vi "ELVIS III v1.0 Configure UART.vi"(7 "Reserve?":bool, 8 "error in (no error)":errorcluster, 10 "VISA resource name in":refnum<visa-resource-name>, 11 "myRIO FPGA Ref":T1) -> (0 "error out":errorcluster)   [LabVIEW 2021]
uses:
  <vilib>/myRIO/Common/Instrument Driver Framework/Utilities/typedefs/Generic FPGA Reference.ctl
  <vilib>/myRIO/Common/Instrument Driver Framework/ELVIS III v1.0/UART/typedefs/ELVIS III v1.0 UART Channels FPGA Reference.ctl
  <vilib>/rvi/errors/niLvFpgaAdjustHostInterfaceError.vi
  <vilib>/rvi/interface/nirviReadWriteControl/nirviReadWriteControl.xnode
  <vilib>/rvi/interface/Simulation/niFpgaSimulationCallBeginRW.vi
  NiFpgaLv.dll
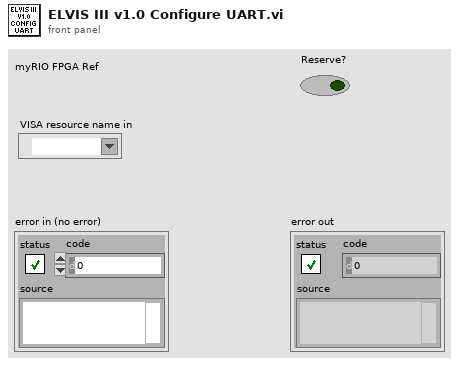
[diagram p1: front panel]
types:
  T1 = typedef "Generic FPGA Reference.ctl" = refnum<k20>
  T2 = typedef "ELVIS III v1.0 UART Channels FPGA Reference.ctl" = refnum<k20>
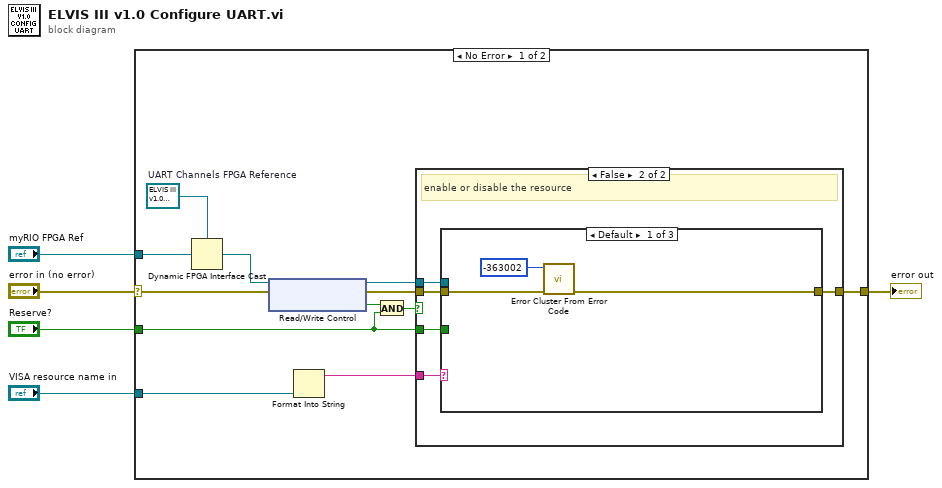
[diagram p0: block diagram]
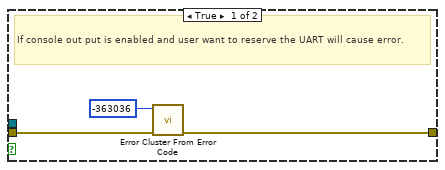
[diagram p2: hidden frame]
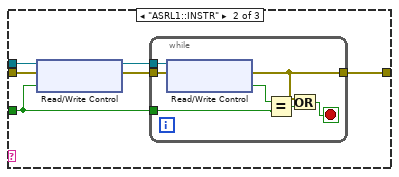
[diagram p3: hidden frame]
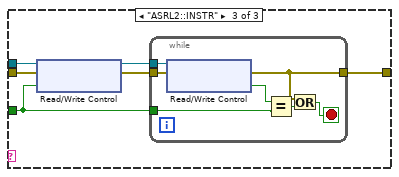
[diagram p4: hidden frame]
diagram:
  n1 = case shown="No Error" "error in (no error)" {
    selector: "error in (no error)" -> [w11 w55]
    tunnel: "myRIO FPGA Ref" -> [w17 _]
    tunnel: "VISA resource name in" -> [w9 _]
    tunnel: [w14 w55] -> w3
    tunnel: "Reserve?" -> [w7 _]
    frame No Error {
      w16 = T2 refnum  # UART Channels FPGA Reference
      n2 = Dynamic FPGA Interface Cast(Session In=w16, Type=w17) -> (Session Out=w13:T2)
      n3 = xnode "Read/Write Control"("FPGA VI Reference In"=w13, "error in"=w11) -> ("FPGA VI Reference Out"=w12:T2, "error out"=w10:errorcluster, "CONSOLE.ENA"=w8:bool)
      n4 = Format Into String(w9) -> (resulting string=w15:string)  [unwired: 3 in, 1 out]
      n5 = And(x=w8, y=w7) -> (x .and. y?=w6:bool)
      n6 = case shown="False" w6 {
        tunnel: w15 -> [_ w25]
        tunnel: [w18 w24] -> w14
        tunnel: w7 -> [_ w23]
        tunnel: w12 -> [_ w22]
        tunnel: w10 -> [w19 w21]
        frame True {
          # "If console out put is enabled and user want to reserve the UART will cause error."
          n7 = call <vilib>:"Error Cluster From Error Code.vi"("error in (no error)"=w19, "error code (0)"=-363036) -> ("error out"=w18:errorcluster)  [unwired: 7 in]
        }
        frame False {
          # "enable or disable the resource"
          n8 = case shown="Default" w25 {
            tunnel: w21 -> [w27 w34 w47]
            tunnel: [w26 w30 w43] -> w24
            tunnel: w23 -> [_ w31 w44]
            tunnel: w22 -> [_ w33 w46]
            frame Default {
              n9 = call <vilib>:"Error Cluster From Error Code.vi"("error in (no error)"=w27, "error code (0)"=-363002) -> ("error out"=w26:errorcluster)  [unwired: 7 in]
            }
            frame "ASRL1::INSTR" {
              n10 = xnode "Read/Write Control"("FPGA VI Reference In"=w33, "error in"=w34, "UART.A.ENA"=w31) -> ("FPGA VI Reference Out"=w32:T2, "error out"=w29:errorcluster)
              n11 = while {
                tunnel: [w40] -> w30
                tunnel: w32 -> [w37]
                tunnel: w31 -> [w36]
                tunnel: w29 -> [w35]
                stop <- w38 stop-if-true
                n12 = xnode "Read/Write Control"("FPGA VI Reference In"=w37, "error in"=w35) -> ("error out"=w40:errorcluster, "UART.A.ENA"=w41:bool)  [unwired: 1 out]
                n13 = Equal?(x=w41, y=w36) -> (x = y?=w39:bool)
                n14 = Or(x=w40, y=w39) -> (x .or. y?=w38:bool)
              }
            }
            frame "ASRL2::INSTR" {
              n15 = xnode "Read/Write Control"("FPGA VI Reference In"=w46, "error in"=w47, "UART.B.ENA"=w44) -> ("FPGA VI Reference Out"=w45:T2, "error out"=w42:errorcluster)
              n16 = while {
                tunnel: [w53] -> w43
                tunnel: w45 -> [w50]
                tunnel: w44 -> [w49]
                tunnel: w42 -> [w48]
                stop <- w51 stop-if-true
                n17 = xnode "Read/Write Control"("FPGA VI Reference In"=w50, "error in"=w48) -> ("error out"=w53:errorcluster, "UART.B.ENA"=w54:bool)  [unwired: 1 out]
                n18 = Equal?(x=w54, y=w49) -> (x = y?=w52:bool)
                n19 = Or(x=w53, y=w52) -> (x .or. y?=w51:bool)
              }
            }
          }
        }
      }
    }
    frame Error {
    }
  }
  "error out" <- w3
